vi "Shutdown.vi"(8 "error in":errorcluster, 11 "PAS in":refnum<class "PAS.lvclass">) -> (0 "error out":errorcluster, 3 "PAS out":refnum<class "PAS.lvclass">)   [LabVIEW 2014, in "PAS.lvclass"]
doc: "Shutoff the DC power which will control all outputs, close all references to DAQmx tasks and shutoff the laser AO."
uses:
  PAS.lvclass
  Instrument/Instrument.lvclass
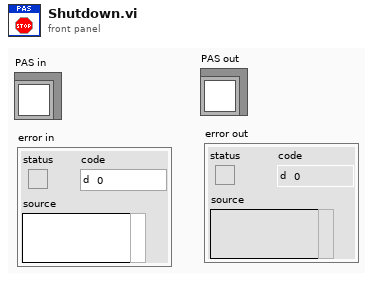
[diagram p1: front panel]
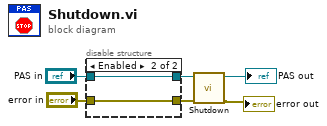
[diagram p0: block diagram]
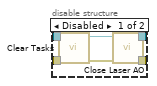
[diagram p2: hidden frame]
diagram:
  n1 = disable-structure shown="Enabled" {
    disable-tunnel: [w10 w14] -> w5
    disable-tunnel: [w9 w13] -> w4
    disable-tunnel: "PAS in" -> [w8 w14]
    disable-tunnel: "error in" -> [w7 w13]
    frame Disabled {
      n2 = call "Clear Tasks.vi"("error in"=w7, "PAS in"=w8) -> ("error out"=w11:errorcluster, "PAS out"=w12:refnum<class "PAS.lvclass">)  [unwired: 8 in]
      n3 = call-dynamic "Close Laser AO.vi"("error in"=w11, "PAS in"=w12) -> ("error out"=w9:errorcluster, "PAS out"=w10:refnum<class "PAS.lvclass">)  [unwired: 8 in]
    }
    frame Enabled {
    }
  }
  n4 = call-parent "Shutdown.vi"("error in"=w4, "Instrument in"=w5) -> ("error out"=→"error out":errorcluster, "Instrument out"=→"PAS out":refnum<class "PAS.lvclass">)  [unwired: 8 in]
